vi "Set State.vi"(7 "VI Ref":refnum<vi>, 8 "Error":errorcluster, 9 "State":T1(ring)=enum."Standard", 11 "(FP)":refnum<class "DecFrame_FP.lvclass">) -> (0 "Error Out":errorcluster, 3 "(FP) Out":refnum<class "DecFrame_FP.lvclass">, 5 "VI Ref":refnum<vi>)   [LabVIEW 2016, in "DecFrame_FP.lvclass"]
uses:
  DecFrame_FP.lvclass
  TypeDefs_Utility/ENUM RB_Pos_Quadrant Position.ctl
  TypeDefs_Utility/Cluster_Pos_Top Left position.ctl
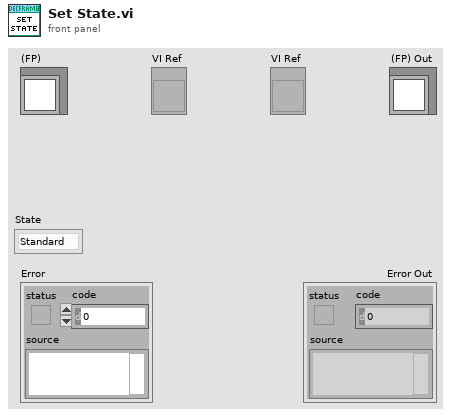
[diagram p1: front panel]
types:
  T1 = enum32{"Invalid", "Standard", "Closed", "Hidden", "Minimized", "Maximized"}
  T2 = typedef "Cluster_Pos_Top Left position.ctl" = cluster{"Left":i16, "Top":i16}
  T3 = typedef "ENUM RB_Pos_Quadrant Position.ctl" = enum32{"LFT-TOP", "MID-TOP", "RGT-TOP", "LFT-CTR", "MID-CTR", "RGT-CTR", "LFT-BOT", "MID-BOT", "RGT-BOT"}
  T4 = enum32{"invalid app kind", "Development System", "Run Time System", "Student Edition", "Embedded LabVIEW", "Evaluation", "Custom"}
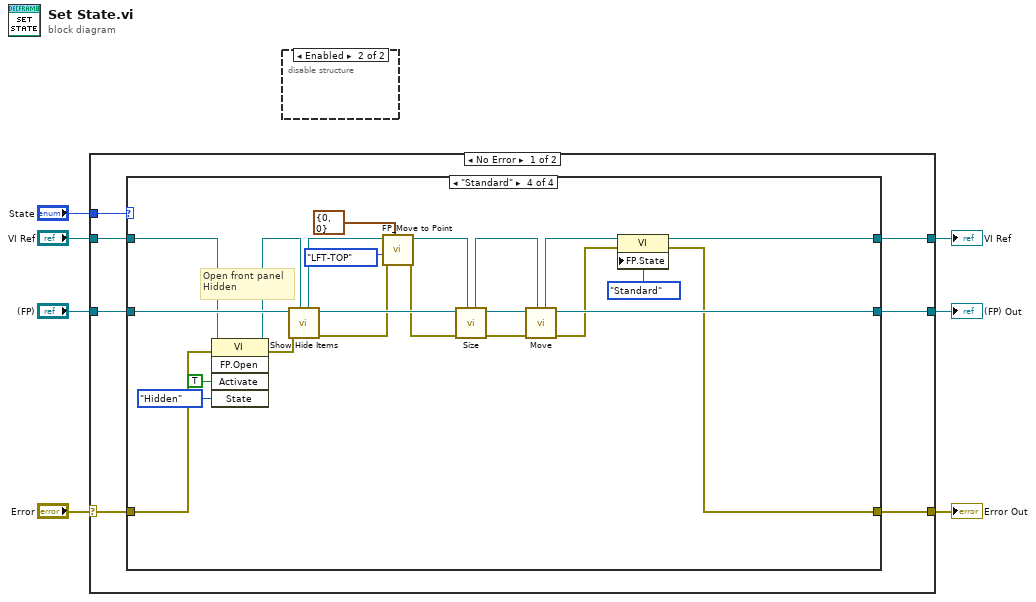
[diagram p0: block diagram]
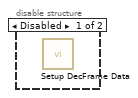
[diagram p2: hidden frame]
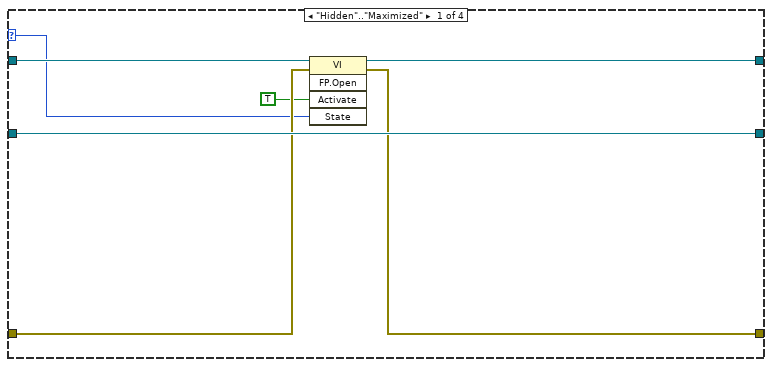
[diagram p3: hidden frame]
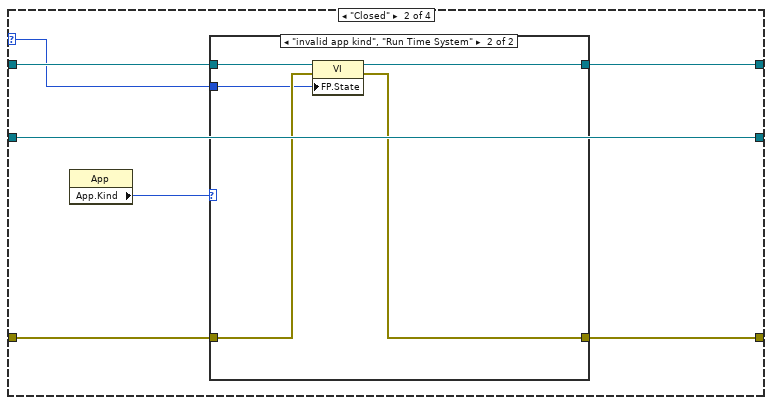
[diagram p4: hidden frame]
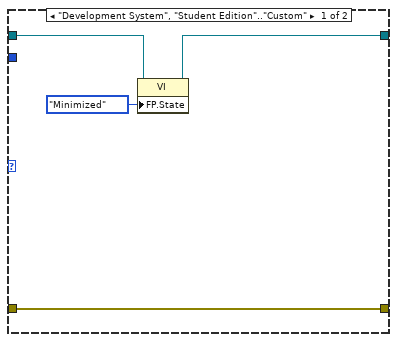
[diagram p5: hidden frame]
diagram:
  n1 = case shown="No Error" "Error" {
    selector: "Error" -> [w11 w66]
    tunnel: [w8 w66] -> w6
    tunnel: [w9 w65] -> w4
    tunnel: "(FP)" -> [w12 w65]
    tunnel: "VI Ref" -> [w13 w64]
    tunnel: [w10 w64] -> w2
    tunnel: "State" -> [w14 _]
    frame No Error {
      n2 = case shown="\"Standard\"" w14 {
        selector: w14 -> [w15 w23 _ _]
        tunnel: w13 -> [w20 w27 w39 w54]
        tunnel: w12 -> [w21 w28 w40 w57]
        tunnel: w11 -> [w18 w25 w38 w52]
        tunnel: [w19 w26 w39 w42] -> w10
        tunnel: [w21 w28 w40 w48] -> w9
        tunnel: [w17 w24 w38 w44] -> w8
        frame "Hidden".."Maximized" {
          n3 = invoke class="VI" method="FP.Open"(reference=w20, error in=w18, "Activate"=TRUE ("Activate?"), "State"=w15) -> (reference out=w19:refnum<vi>, error out=w17:errorcluster)  [unwired: 1 in, 3 out]
        }
        frame "Closed" {
          n4 = property class="App"() -> ("App.Kind"=w22:T4)  [unwired: 2 in, 2 out]
          n5 = case shown="\"invalid app kind\", \"Run Time System\"" w22 {
            tunnel: w27 -> [w31 w37]
            tunnel: [w30 w36] -> w26
            tunnel: w25 -> [w32 w35]
            tunnel: [w32 w34] -> w24
            tunnel: w23 -> [_ w33]
            frame "Development System", "Student Edition".."Custom" {
              n6 = property class="VI"(reference=w31, "FP.State"=T1."Minimized" ("Front Panel Window:State")) -> (reference out=w30:refnum<vi>)  [unwired: 1 in, 1 out]
            }
            frame "invalid app kind", "Run Time System" {
              n7 = property class="VI"(reference=w37, error in=w35, "FP.State"=w33) -> (reference out=w36:refnum<vi>, error out=w34:errorcluster)
            }
          }
        }
        frame "Invalid" {
        }
        frame "Standard" {
          # "Open front panel\nHidden"
          n8 = invoke class="VI" method="FP.Open"(reference=w54, error in=w52, "Activate"=TRUE ("Activate?"), "State"=T1."Hidden") -> (reference out=w53:refnum<vi>, error out=w51:errorcluster)  [unwired: 1 in, 3 out]
          n9 = call-dynamic "Show Hide Items.vi"("VI Ref"=w53, "Error"=w51, "(FP)"=w57) -> ("Error Out"=w41:errorcluster, "(FP) Out"=w63:refnum<class "DecFrame_FP.lvclass">, "VI Ref Out"=w62:refnum<vi>)  [unwired: 6 in]
          n10 = call "FP_Move to Point.vi"("Target Point"=T2 {"Left"=0, "Top"=0}, "Error"=w41, "FP Position"=ENUM_RB_Pos_Quadrant_Position."LFT-TOP", "VI"=w62) -> ("Error Out"=w58:errorcluster, "VI Out"=w61:refnum<vi>)  [unwired: 6 in]
          n11 = call "Size.vi"("VI Ref"=w61, "Error"=w58, "DecFrame_FP"=w63) -> ("Error Out"=w47:errorcluster, "DecFrame_FP Out"=w49:refnum<class "DecFrame_FP.lvclass">, "VI Out"=w46:refnum<vi>)  [unwired: 6 in]
          n12 = call "Move.vi"("VI Ref"=w46, "Error"=w47, "DecFrame_FP"=w49) -> ("Error Out"=w45:errorcluster, "DecFrame_FP Out"=w48:refnum<class "DecFrame_FP.lvclass">, "VI Out"=w43:refnum<vi>)  [unwired: 6 in]
          n13 = property class="VI"(reference=w43, error in=w45, "FP.State"=T1."Standard" ("Front Panel Window:State")) -> (reference out=w42:refnum<vi>, error out=w44:errorcluster)
        }
      }
    }
    frame Error {
    }
  }
  "Error Out" <- w6
  "(FP) Out" <- w4
  "VI Ref" <- w2
  n14 = disable-structure shown="Enabled" {
    frame Disabled {
      n15 = call-dynamic "Setup DecFrame Data.vi"() -> ()  [unwired: 10 in, 2 out]
    }
    frame Enabled {
    }
  }
